vi "ProjFile_Write File.vi"(7 "LV Project Path":path, 8 "error in":errorcluster, 9 "Resource Data":T1, 10 "Project Data":T4, 11 "file path (use dialog)":path) -> (0 "error out":errorcluster, 3 "path":path)   [LabVIEW 2013, in "SET Project Data.lvlib"]
doc: "ProjFile_Write File.vi\n\nWrite Project Data and Resource data to a SET Project File (specified by \"file path\" input)."
uses:
  SET Project Data.lvlib
  Types/ProjFile_Project Data.ctl
  Types/ProjFile_Menu Data.ctl
  Types/ProjFile_VI Data.ctl
  Types/ProjFile_GObject Data.ctl
  Types/ProjFile_Resources Data.ctl
  Types/ProjFile_Language Entry.ctl
  Types/ProjFile_Resource Entry.ctl
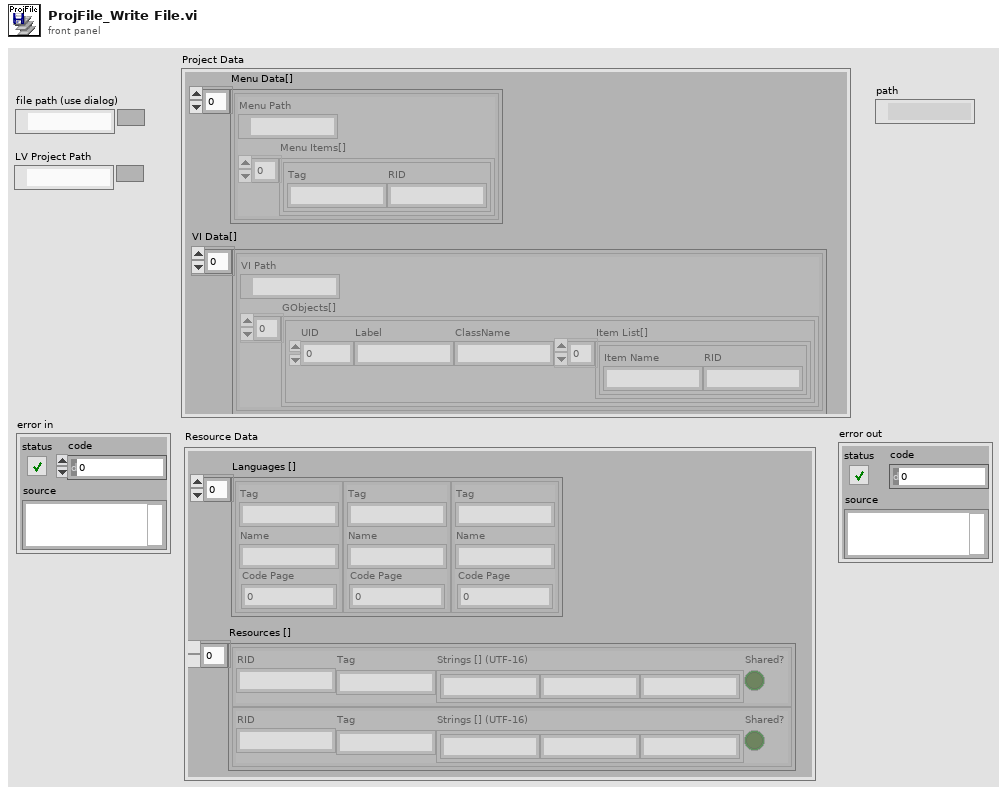
[diagram p1: front panel]
types:
  T1 = typedef "SET Project Data.lvlib/ProjFile_Resources Data.ctl" = cluster{"Languages []":T2[], "Resources []":T3[]}
  T2 = typedef "SET Project Data.lvlib/ProjFile_Language Entry.ctl" = cluster{"Tag":string, "Name":string, "Code Page":u16}
  T3 = typedef "SET Project Data.lvlib/ProjFile_Resource Entry.ctl" = cluster{"RID":string, "Tag":string, "Strings [] (UTF-16)":string[], "Shared?":bool}
  T4 = typedef "SET Project Data.lvlib/ProjFile_Project Data.ctl" = cluster{"Menu Data[]":T5[], "VI Data[]":T6[]}
  T5 = typedef "SET Project Data.lvlib/ProjFile_Menu Data.ctl" = cluster{"Menu Path":path, "Menu Items[]":cluster{"Tag":string, "RID":string}[]}
  T6 = typedef "SET Project Data.lvlib/ProjFile_VI Data.ctl" = cluster{"VI Path":path, "GObjects[]":T7[]}
  T7 = typedef "SET Project Data.lvlib/ProjFile_GObject Data.ctl" = cluster{"UID":i32, "Label":string, "ClassName":string, "Item List[]":cluster{"Item Name":string, "RID":string}[]}
  T8 = enum16{"open", "replace", "create", "open or create", "replace or create", "replace or create with confirmation"}
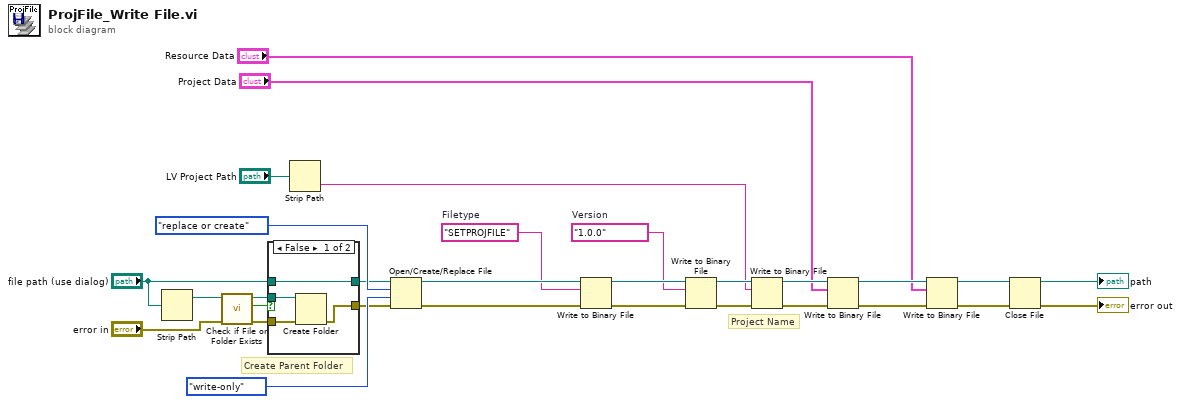
[diagram p0: block diagram]
diagram:
  w23 = "1.0.0"  # Version
  w26 = "SETPROJFILE"  # Filetype
  # "Create Parent Folder"
  # "Project Name"
  n1 = Strip Path(path="file path (use dialog)") -> (stripped path=w8:path)  [unwired: 1 out]
  n2 = call <vilib>:"Check if File or Folder Exists.vi"("error in (no error)"="error in", "path"=w8) -> ("error out"=w3:errorcluster, "file or folder exists?"=w6:bool, "dup path"=w4:path)  [unwired: 7 in]
  n3 = case shown="False" w6 {
    tunnel: "file path (use dialog)" -> [w31 w36]
    tunnel: w4 -> [w34 _]
    tunnel: w3 -> [w33 w35]
    tunnel: [w32 w35] -> w2
    tunnel: [w31 w36] -> w1
    frame False {
      n4 = Create Folder(path (use dialog)=w34, error in=w33) -> (error out=w32:errorcluster)  [unwired: 1 in, 2 out]
    }
    frame True {
    }
  }
  n5 = Strip Path(path="LV Project Path") -> (name=w15:string)  [unwired: 1 out]
  n6 = Open/Create/Replace File(file path (use dialog)=w1, error in=w2, operation (0:open)=T8."replace or create", access (0:read/write)=enum16{"read/write", "read-only", "write-only"}."write-only") -> (refnum out=w28:refnum<file>, error out=w27:errorcluster)  [unwired: 2 in, 1 out]
  n7 = Write to Binary File(file (use dialog)=w28, data=w26, error in=w27) -> (refnum out=w25:refnum<file>, error out=w24:errorcluster)  [unwired: 3 in, 1 out]
  n8 = Write to Binary File(file (use dialog)=w25, data=w23, error in=w24) -> (refnum out=w22:refnum<file>, error out=w21:errorcluster)  [unwired: 3 in, 1 out]
  n9 = Write to Binary File(file (use dialog)=w22, data=w15, error in=w21) -> (refnum out=w20:refnum<file>, error out=w19:errorcluster)  [unwired: 3 in, 1 out]
  n10 = Write to Binary File(file (use dialog)=w20, data="Project Data", error in=w19) -> (refnum out=w13:refnum<file>, error out=w12:errorcluster)  [unwired: 3 in, 1 out]
  n11 = Write to Binary File(file (use dialog)=w13, data="Resource Data", error in=w12) -> (refnum out=w10:refnum<file>, error out=w11:errorcluster)  [unwired: 3 in, 1 out]
  n12 = Close File(refnum=w10, error in=w11) -> (path=→"path":path, error out=→"error out":errorcluster)
